vi "Colour Image to Numpy Array.vi"(8 "error in (no error)":errorcluster, 11 "Refnum in":T1) -> (0 "error out":errorcluster, 3 "Array":u8[][][](array[numeric]))   [LabVIEW 2025, in "Coin Analyser.lvclass"]
doc: "OpenCV can take an image as a 3d numpy array.\n\nThis converts a colour image to that format - with 3 dimensions for each colour plane."
uses:
  Coin Analyser.lvclass
  <vilib>/vision/Image Controls.llb/IMAQ Image.ctl
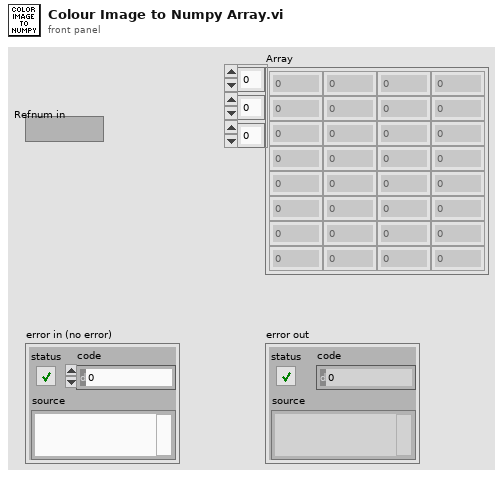
[diagram p1: front panel]
types:
  T1 = typedef "IMAQ Image.ctl" = refnum<image>
  T2 = enum16{"big-endian, network order", "native, host order", "little-endian"}
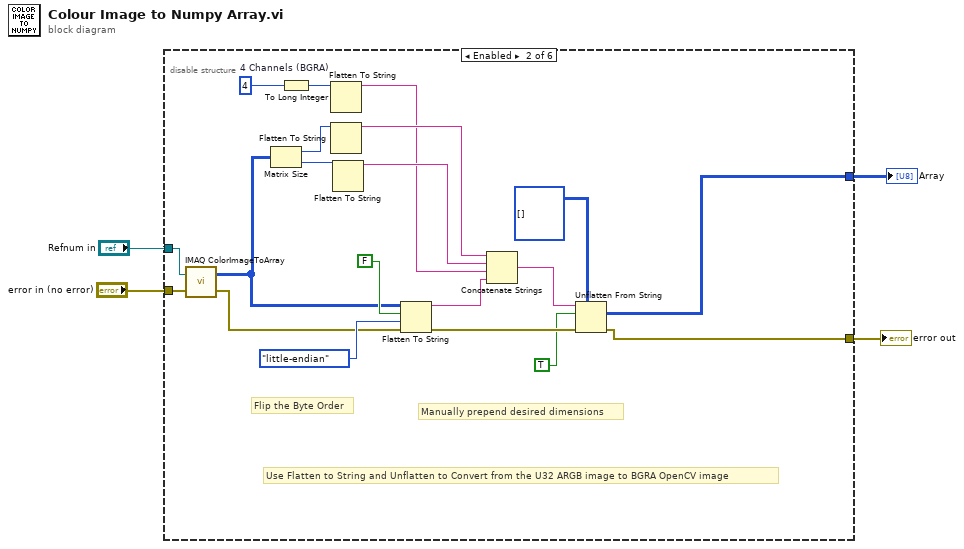
[diagram p0: block diagram]
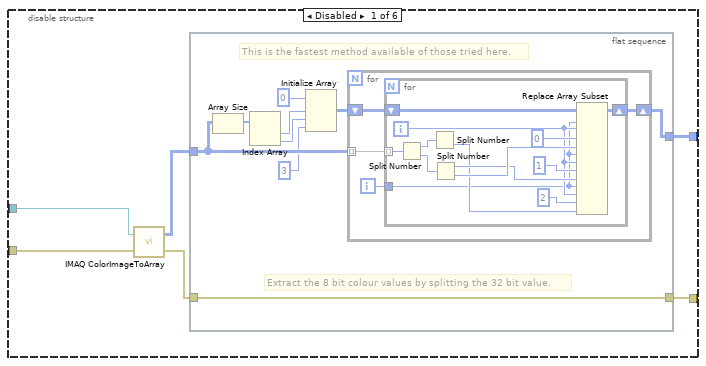
[diagram p2: hidden frame]
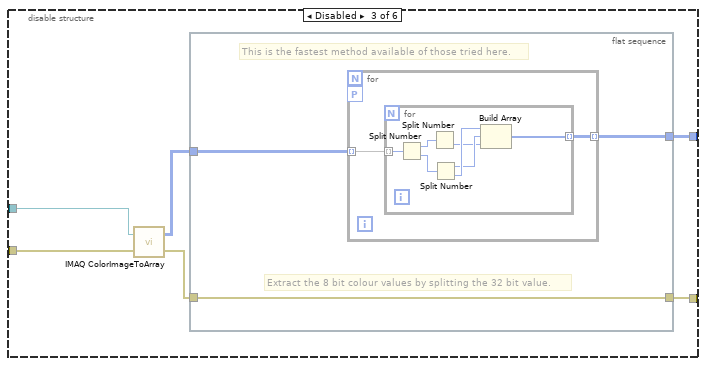
[diagram p3: hidden frame]
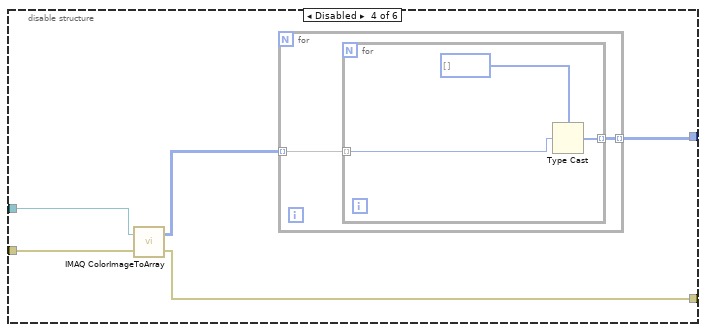
[diagram p4: hidden frame]
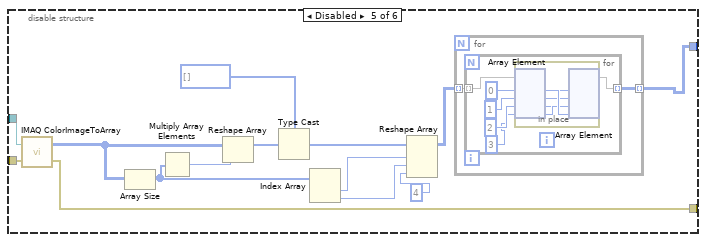
[diagram p5: hidden frame]
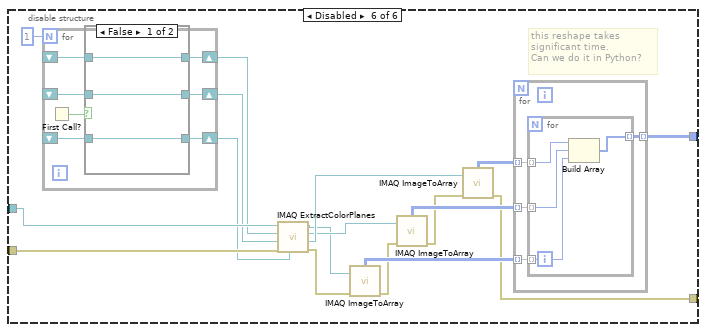
[diagram p6: hidden frame]
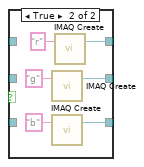
[diagram p7: hidden frame]
diagram:
  n1 = disable-structure shown="Enabled" {
    disable-tunnel: "Refnum in" -> [w10 w41 w62 w79 w98 w126]
    disable-tunnel: [w6 w37 w58 w78 w97 w115] -> w3
    disable-tunnel: "error in (no error)" -> [w9 w42 w61 w77 w96 w127]
    disable-tunnel: [w7 w38 w59 w75 w88 w119] -> w1
    frame Disabled {
      n2 = call "IMAQ ColorImageToArray"("Image"=w10, "error in (no error)"=w9) -> ("Image Pixels (U32)"=w8:u32[][], "error out"=w5:errorcluster)  [unwired: 2 in, 1 out]
      n3 = flat-sequence {
        tunnel: w8 -> [w18]
        tunnel: [w11] -> w7
        tunnel: [w19] -> w6
        tunnel: w5 -> [w19]
        frame #0 {
          # "Extract the 8 bit colour values by splitting the 32 bit value."
          # "This is the fastest method available of those tried here."
          n4 = Array Size(array=w18) -> (size(s)=w17:i32[])
          n5 = Index Array(array=w17) -> (element #1=w16:i32, element #2=w15:i32)  [unwired: 2 in]
          n6 = Initialize Array(u8 0 ("dimension size"), w16, w15, 3 ("dimension size")) -> (w12:u8[][][])
          n7 = for {
            tunnel: w18 -> [w23] mode=indexing
            shift-right: [w21] -> w11
            shift-left: w12 -> [w22]
            i -> [w20]
            n8 = for {
              tunnel: w23 -> [w36] mode=indexing
              shift-right: [w32] -> w21
              shift-left: w22 -> [w33]
              tunnel: w20 -> [w24]
              i -> [w25]
              n9 = Split Number(x=w36) -> (hi(x)=w35:u16, lo(x)=w34:u16)
              n10 = Split Number(x=w35) -> (lo(x)=w29:u8)  [unwired: 1 out]
              n11 = Split Number(x=w34) -> (hi(x)=w30:u8, lo(x)=w31:u8)
              n12 = Replace Array Subset(array=w33, new element #1=w31, index (dim 0) #1=w24, index (dim 1) #1=w25, index (dim 2) #1=0 ("index (page)"), new element #2=w30, index (dim 0) #2=w24, index (dim 1) #2=w25, index (dim 2) #2=1 ("index (page)"), new element #3=w29, index (dim 0) #3=w24, index (dim 1) #3=w25, index (dim 2) #3=2 ("index (page)")) -> (w32:u8[][][])
            }
          }
        }
      }
    }
    frame Enabled {
      w43 = 4  # 4 Channels (BGRA)
      # "Use Flatten to String and Unflatten to Convert from the U32 ARGB image to BGRA OpenCV image"
      # "Flip the Byte Order"
      # "Manually prepend desired dimensions"
      n13 = call "IMAQ ColorImageToArray"("Image"=w41, "error in (no error)"=w42) -> ("Image Pixels (U32)"=w40:u32[][], "error out"=w39:errorcluster)  [unwired: 2 in, 1 out]
      n14 = Matrix Size(0:w40) -> (1:w50:i32, 2:w49:i32)
      n15 = To Long Integer(number=w43) -> (32bit integer=w51:i32)
      n16 = Flatten To String(anything=w51) -> (data string=w54:string)  [unwired: 3 in, 2 out]
      n17 = Flatten To String(anything=w50) -> (data string=w55:string)  [unwired: 3 in, 2 out]
      n18 = Flatten To String(anything=w49) -> (data string=w56:string)  [unwired: 3 in, 2 out]
      n19 = Flatten To String(anything=w40, prepend array or string size? (T)=FALSE, byte order (0:big-endian, network order)=T2."little-endian", error in (no error)=w39) -> (data string=w52:string, error out=w48:errorcluster)  [unwired: 1 out]
      n20 = Concatenate Strings(w55, w56, w54, w52) -> (w53:string)
      n21 = Unflatten From String(type=u8[][][] [] ("Array"), binary string=w53, data includes array or string size? (T)=TRUE, error in (no error)=w48) -> (value=w38:u8[][][], error out=w37:errorcluster)  [unwired: 1 in, 1 out]
    }
    frame Disabled {
      n22 = call "IMAQ ColorImageToArray"("Image"=w62, "error in (no error)"=w61) -> ("Image Pixels (U32)"=w60:u32[][], "error out"=w57:errorcluster)  [unwired: 2 in, 1 out]
      n23 = flat-sequence {
        tunnel: w60 -> [w65]
        tunnel: [w64] -> w59
        tunnel: [w63] -> w58
        tunnel: w57 -> [w63]
        frame #0 {
          # "Extract the 8 bit colour values by splitting the 32 bit value."
          # "This is the fastest method available of those tried here."
          n24 = for {
            tunnel: w65 -> [w67] mode=indexing
            tunnel: [w66] -> w64 mode=indexing
            workers-P: _ -> [_]
            n25 = for {
              tunnel: w67 -> [w74] mode=indexing
              tunnel: [w71] -> w66 mode=indexing
              n26 = Split Number(x=w74) -> (hi(x)=w73:u16, lo(x)=w72:u16)
              n27 = Split Number(x=w73) -> (lo(x)=w68:u8)  [unwired: 1 out]
              n28 = Split Number(x=w72) -> (hi(x)=w69:u8, lo(x)=w70:u8)
              n29 = Build Array(w70, w69, w68) -> (w71:u8[])
            }
          }
        }
      }
    }
    frame Disabled {
      n30 = call "IMAQ ColorImageToArray"("Image"=w79, "error in (no error)"=w77) -> ("Image Pixels (U32)"=w76:u32[][], "error out"=w78:errorcluster)  [unwired: 2 in, 1 out]
      n31 = for {
        tunnel: w76 -> [w81] mode=indexing
        tunnel: [w80] -> w75 mode=indexing
        n32 = for {
          tunnel: w81 -> [w84] mode=indexing
          tunnel: [w83] -> w80 mode=indexing
          n33 = Type Cast(type=u8[] [] ("Array"), x=w84) -> (*(type *) &x=w83:u8[])
        }
      }
    }
    frame Disabled {
      n34 = call "IMAQ ColorImageToArray"("Image"=w98, "error in (no error)"=w96) -> ("Image Pixels (U32)"=w93:u32[][], "error out"=w97:errorcluster)  [unwired: 2 in, 1 out]
      n35 = Array Size(array=w93) -> (size(s)=w91:i32[])
      n36 = Multiply Array Elements(1:w91) -> (0:w90:i32)
      n37 = Reshape Array(w93, w90) -> (w92:u32[])
      n38 = Type Cast(type=u8[] [], x=w92) -> (*(type *) &x=w95:u8[])
      n39 = Index Array(array=w91) -> (element #1=w86:i32, element #2=w85:i32)  [unwired: 2 in]
      n40 = Reshape Array(w95, w86, w85, 4 ("dimension size")) -> (w89:u8[][][])
      n41 = for {
        tunnel: w89 -> [w100] mode=indexing
        tunnel: [w99] -> w88 mode=indexing
        n42 = for {
          tunnel: w100 -> [w106] mode=indexing
          tunnel: [w105] -> w99 mode=indexing
          n43 = in-place {
            n44 = in-place-array #1(w106, 0, 1, 2, 3) -> (w110:u8, w108:u8, w107:u8, w109:u8)
            n45 = in-place-array #1(w107, w108, w109, w110) -> (w105:u8[])  [unwired: 4 out]
          }
        }
      }
    }
    frame Disabled {
      # "this reshape takes\nsignificant time.\nCan we do it in Python?"
      n46 = for {
        N: 1 -> [_]
        shift-right: [w140] -> w112
        shift-left: _ -> [w138]
        shift-right: [w141] -> w113
        shift-left: _ -> [w137]
        shift-right: [w142] -> w114
        shift-left: _ -> [w136]
        n47 = First Call?() -> (First Call?: T/F=w139:bool)
        n48 = case shown="False" w139 {
          tunnel: [w143 w151] -> w142
          tunnel: [w144 w150] -> w141
          tunnel: [w145 w149] -> w140
          tunnel: w138 -> [w145 _]
          tunnel: w137 -> [w144 _]
          tunnel: w136 -> [w143 _]
          frame False {
          }
          frame True {
            n49 = call "IMAQ Create"("Image Name"="g") -> ("New Image"=w150:T1)  [unwired: 4 in, 1 out]
            n50 = call "IMAQ Create"("Image Name"="b") -> ("New Image"=w151:T1)  [unwired: 4 in, 1 out]
            n51 = call "IMAQ Create"("Image Name"="r") -> ("New Image"=w149:T1)  [unwired: 4 in, 1 out]
          }
        }
      }
      n52 = call "IMAQ ExtractColorPlanes"("Blue or Luma or Val or Inten Plane"=w114, "error in (no error)"=w127, "Green or Sat Plane"=w113, "Red or Hue Plane"=w112, "Image Src"=w126) -> ("error out"=w118:errorcluster, "Blue or Luma or Val or Inten Plane out"=w125:T1, "Green or Sat Plane out"=w124:T1, "Red or Hue Plane out"=w123:T1)  [unwired: 3 in]
      n53 = call "IMAQ ImageToArray"("error in (no error)"=w118, "Image"=w123) -> ("error out"=w117:errorcluster, "Image Pixels (U8)"=w122:u8[][])  [unwired: 2 in, 3 out]
      n54 = call "IMAQ ImageToArray"("error in (no error)"=w117, "Image"=w124) -> ("error out"=w116:errorcluster, "Image Pixels (U8)"=w121:u8[][])  [unwired: 2 in, 3 out]
      n55 = call "IMAQ ImageToArray"("error in (no error)"=w116, "Image"=w125) -> ("error out"=w115:errorcluster, "Image Pixels (U8)"=w120:u8[][])  [unwired: 2 in, 3 out]
      n56 = for {
        tunnel: w122 -> [w131] mode=indexing
        tunnel: w121 -> [w130] mode=indexing
        tunnel: w120 -> [w129] mode=indexing
        tunnel: [w128] -> w119 mode=indexing
        n57 = for {
          tunnel: w131 -> [w135] mode=indexing
          tunnel: w130 -> [w134] mode=indexing
          tunnel: w129 -> [w133] mode=indexing
          tunnel: [w132] -> w128 mode=indexing
          n58 = Build Array(w133, w134, w135) -> (w132:u8[])
        }
      }
    }
  }
  "Array" <- w1
  "error out" <- w3
